vi "RT_position_plus.vi"() -> ()   [LabVIEW 2014]
uses:
  <vilib>/FPGAPlugInAG/cRIO-9068/niLvFpga_Open_cRIO-9068.vi
  <vilib>/rvi/interface/common/dynamic/niFpgaDynamicAddResources.vi
  <vilib>/Utility/error.llb/Error Cluster From Error Code.vi
  <vilib>/rvi/errors/niLvFpgaAdjustHostInterfaceError.vi
  <vilib>/FPGAPlugInAG/Dynamic/niLvFpga_Close_Dynamic.vi
  <vilib>/rvi/interface/nirviOpenFPGA/nirviOpenFPGA.xnode
  FPGA Bitfiles/Motortest_FPGATarget_test6auto_Jx62XASY7Q8.lvbitx
  <vilib>/rvi/interface/nirviReadWriteControl/nirviReadWriteControl.xnode
  <vilib>/rvi/interface/nirviCloseFPGA/nirviCloseFPGA.xnode
  NiFpgaLv.dll
  <vilib>/rvi/interface/Simulation/niFpgaSimulationCallBeginRW.vi
panel:
  out "Duty Cycle":sgl
  in  "Desired Position[Round]":sgl=500.0
  out "Position":cluster{i32[], sgl[]}(graph)
  out "Position[Round]":sgl
  out "Angular Velocity vs. Duty Cycle":cluster{sgl[], sgl[]}(graph)
  in  "Drive Direction":enum8{"Clockwise", "Counterclockwise"}(ring)=enum."Counterclockwise"
  in  "Velocity Interval (uSec)":u32=500000
  in  "stop":bool
  out "Velocity[RPS]":sgl
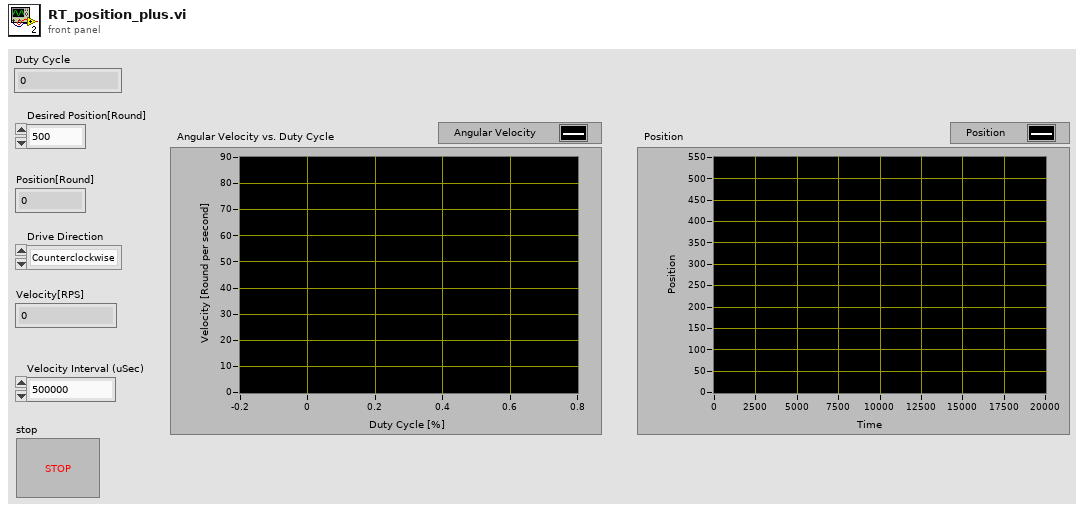
[diagram p1: front panel]
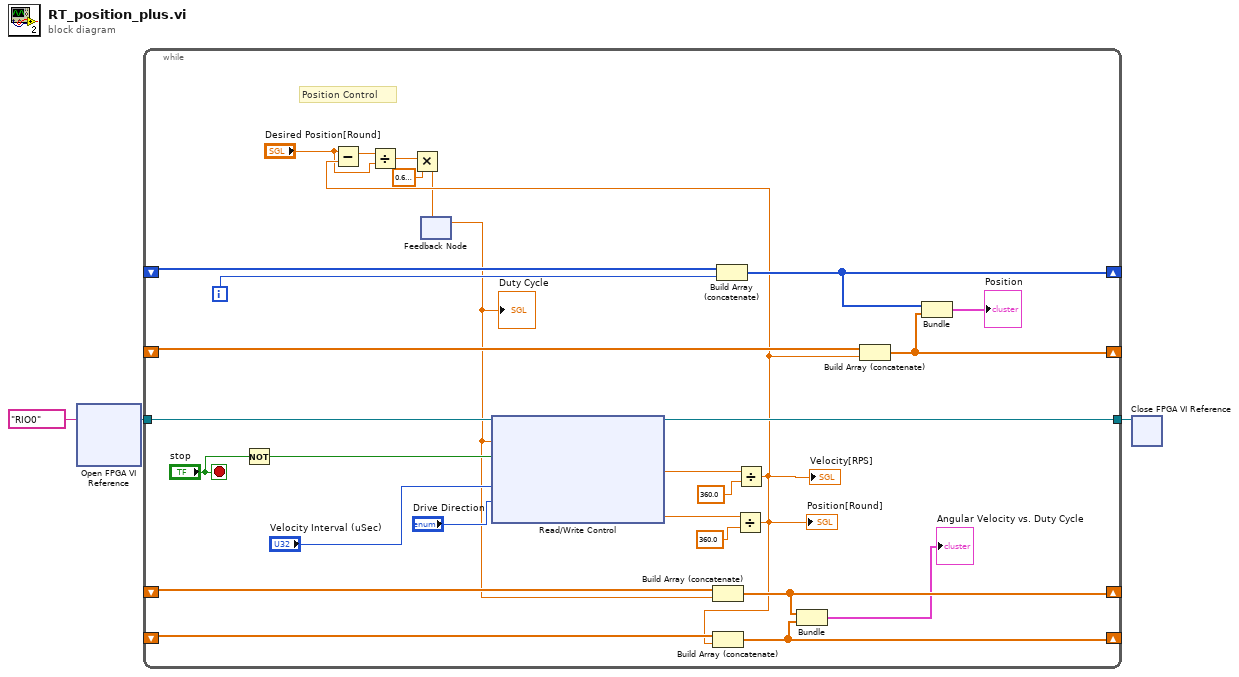
[diagram p0: block diagram]
diagram:
  n1 = xnode "Open FPGA VI Reference"("resource name"=tag "RIO0") -> ("FPGA VI Reference Out"=w2:refnum<k20>)  [unwired: 1 in, 1 out]
  n2 = while {
    tunnel: w2 -> [w32]
    tunnel: [w31] -> w1
    shift-right: [w27] -> _
    shift-left: _ -> [w14]
    shift-right: [w19] -> _
    shift-left: _ -> [w15]
    shift-right: [w20] -> _
    shift-left: _ -> [w21]
    shift-right: [w17] -> _
    shift-left: _ -> [w18]
    i -> [w22]
    stop <- "stop" stop-if-true
    # "Position Control"
    n3 = Not(x="stop") -> (.not. x?=w12:bool)
    n4 = feedback #1() -> (w5:sgl)  [unwired: 1 in]
    "Duty Cycle" <- w5
    n5 = xnode "Read/Write Control"("FPGA VI Reference In"=w32, "duty cycle (periods)"=w5, "Mod1/Motor"=w12, "Velocity Interval (uSec)"="Velocity Interval (uSec)", "Mod1/Drive Direction"="Drive Direction") -> ("FPGA VI Reference Out"=w31:refnum<k20>, "Velocity (Degrees/Second)"=w26:sgl, "Position (Degrees)"=w23:sgl)  [unwired: 1 in, 1 out]
    n6 = Build Array (concatenate)(w14, w5) -> (w27:sgl[])
    n7 = Build Array (concatenate)(w21, w22) -> (w20:i32[])
    n8 = Divide(x=w23, y=sgl 360.0) -> (x/y=w11:sgl)
    "Position[Round]" <- w11
    n9 = Subtract(x="Desired Position[Round]", y=w11) -> (x-y=w10:sgl)
    n10 = Divide(x=w10, y="Desired Position[Round]") -> (x/y=w8:sgl)
    n11 = Multiply(x=w8, y=sgl 0.6) -> (x*y=w6:sgl)
    n12 = feedback-in #1(w6) -> ()
    n13 = Divide(x=w26, y=sgl 360.0) -> (x/y=w13:sgl)
    "Velocity[RPS]" <- w13
    n14 = Build Array (concatenate)(w15, w13) -> (w19:sgl[])
    n15 = Bundle(w27, w19) -> (→"Angular Velocity vs. Duty Cycle":cluster{sgl[], sgl[]})  [unwired: 1 in]
    n16 = Build Array (concatenate)(w18, w11) -> (w17:sgl[])
    n17 = Bundle(w20, w17) -> (→"Position":cluster{i32[], sgl[]})  [unwired: 1 in]
  }
  n18 = xnode "Close FPGA VI Reference"("FPGA VI Reference In"=w1) -> ()  [unwired: 1 in, 1 out]
